vi "FRCts20_WebMethods_Convert_Teams.vi"(8 "error in (no error)":errorcluster, 11 "Team Out":T1) -> (0 "error out":errorcluster, 3 "Universe":T3)   [LabVIEW 2012, in "FRCts20_WebMethods.lvlib"]
uses:
  FRCts20_WebMethods.lvlib
  ESP Engine/source/VI Source/TypeDefs/FRCts20_EspEngine_Universe.ctl
  ESP Engine/source/VI Source/TypeDefs/FRCts20_EspEngine_Team.ctl
  Web Method Public Interface/FRCts20_WebMethods_ctl_singleTeam.ctl
  Web Method Public Interface/FRCts20_WebMethods_ctl_teamIdentifier.ctl
  Backend/source/VI Source/FRCts20_Backend_API/FRCts20_Backend_API_SW.ctl
  Web Method Public Interface/FRCts20_WebMethods_ctl_request.ctl
  Backend/source/VI Source/FRCts20_Backend_API/FRCts20_Backend_API_Status.ctl
  ESP Engine/source/VI Source/TypeDefs/FRCts20_EspEngine_Event.ctl
  Web Method Public Interface/FRCts20_WebMethods_ctl_singleEvent.ctl
  Backend/source/VI Source/FRCts20_Backend_API/FRCts20_Backend_API_TeamRoot.ctl
  Backend/source/VI Source/FRCts20_Backend_API/FRCts20_Backend_API.lvlib
  ESP Engine/source/VI Source/FRCts20_EspEngine.lvlib
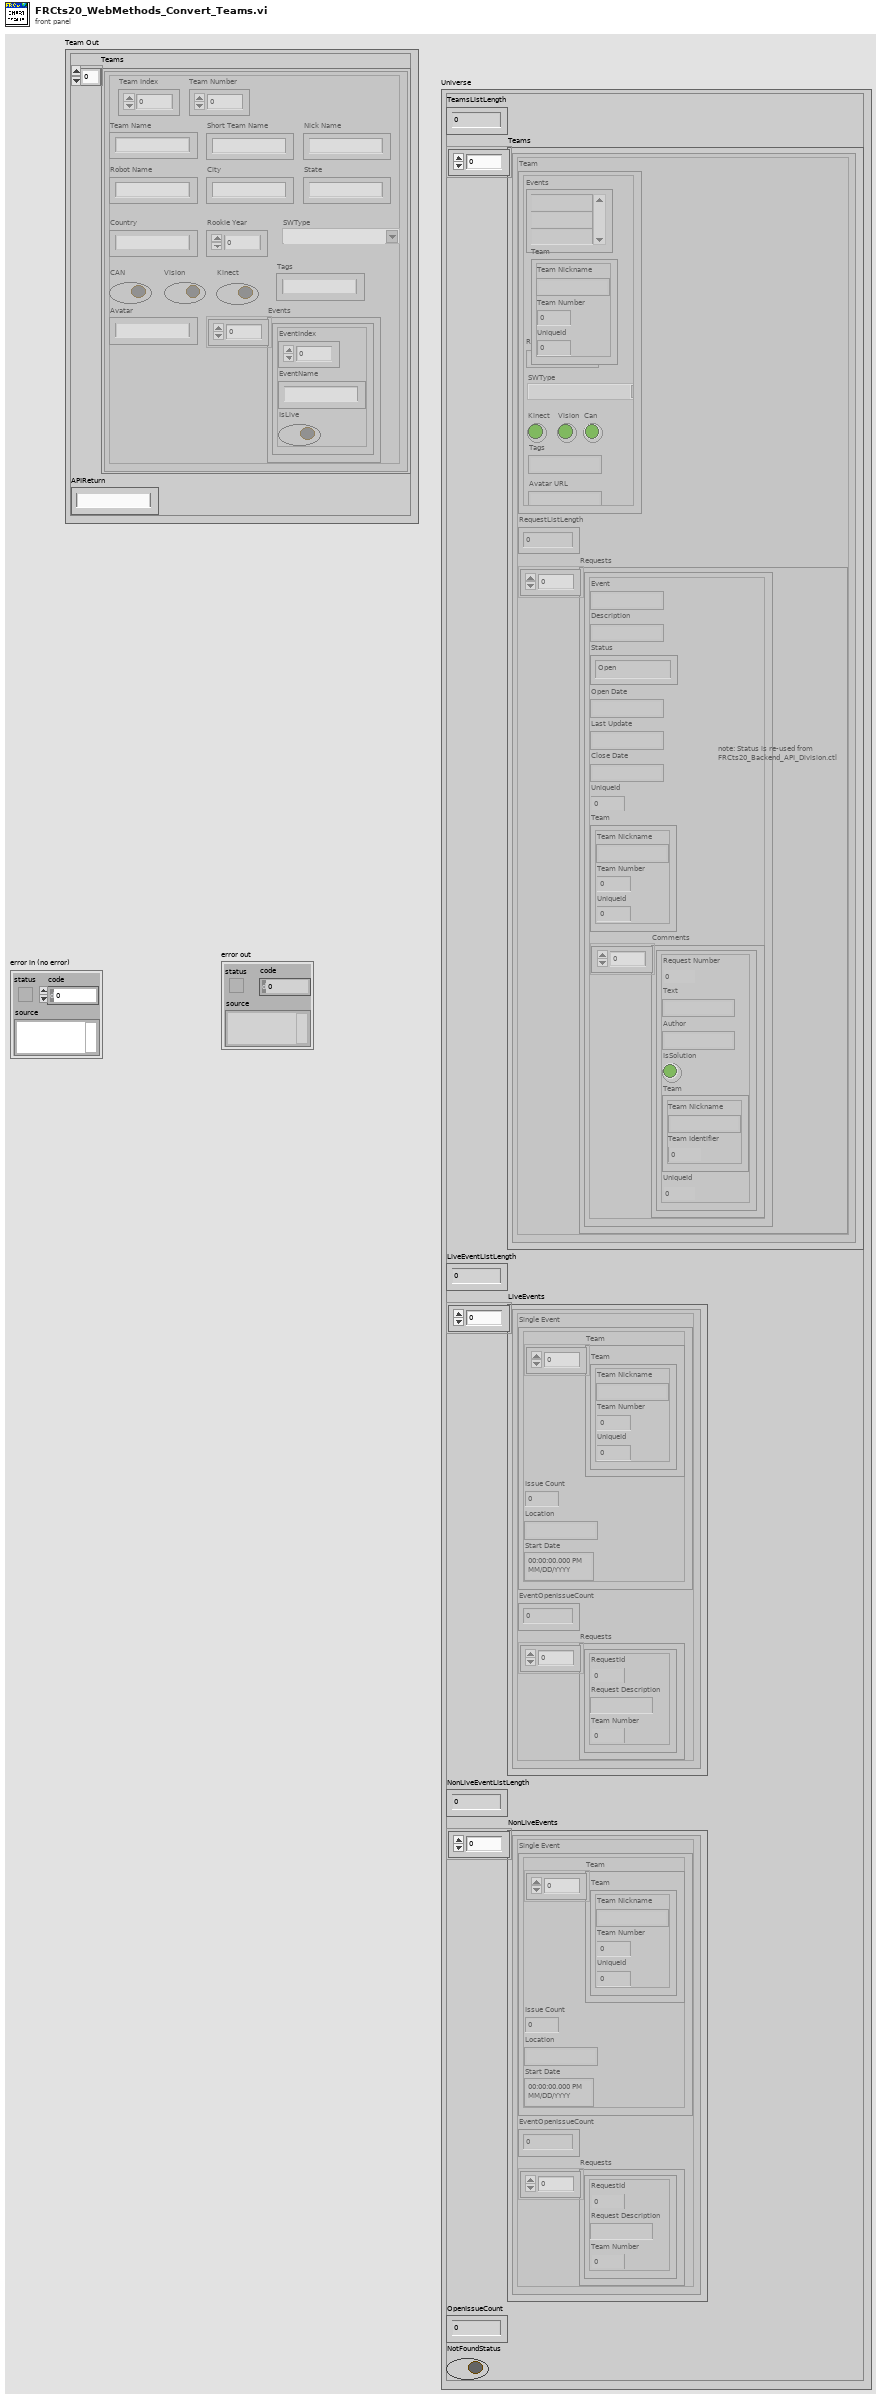
[diagram p1: front panel]
types:
  T1 = typedef "FRCts20_Backend_API.lvlib/FRCts20_Backend_API_TeamRoot.ctl" = cluster{"Teams":cluster{"Team Index":u32, "Team Number":u32, "Team Name":string, "Short Team Name":string, "Nick Name":string, "Robot Name":string, "City":string, "State":string, "Country":string, "Rookie Year":u32, "SWType":T2, "CAN":bool, "Vision":bool, "Kinect":bool, "Tags":string, "Avatar":string, "Events":cluster{"EventIndex":u32, "EventName":string, "IsLive":bool}[]}[], "APIReturn":string}
  T2 = typedef "FRCts20_Backend_API.lvlib/FRCts20_Backend_API_SW.ctl" = string
  T3 = typedef "FRCts20_EspEngine.lvlib/FRCts20_EspEngine_Universe.ctl" = cluster{"TeamsListLength":i16, "Teams":T4[], "LiveEventListLength":i16, "LiveEvents":T9[], "NonLiveEventListLength":i16, "NonLiveEvents":T9[], "OpenIssueCount":i16, "NotFoundStatus":bool}
  T4 = typedef "FRCts20_EspEngine.lvlib/FRCts20_EspEngine_Team.ctl" = cluster{"Team":T5, "RequestListLength":i16, "Requests":T7[]}
  T5 = typedef "FRCts20_WebMethods.lvlib/FRCts20_WebMethods_ctl_singleTeam.ctl" = cluster{"Events":string[], "Robot Name":string, "Kinect":bool, "Vision":bool, "Can":bool, "Tags":string, "Avatar URL":string, "Team":T6, "SWType":T2}
  T6 = typedef "FRCts20_WebMethods.lvlib/FRCts20_WebMethods_ctl_teamIdentifier.ctl" = cluster{"Team Nickname":string, "Team Number ":u32, "UniqueId":u32}
  T7 = typedef "FRCts20_WebMethods.lvlib/FRCts20_WebMethods_ctl_request.ctl" = cluster{"Event":string, "Description":string, "Status":T8, "Open Date":string, "Last Update":string, "Close Date":string, "UniqueId":i32, "Team":cluster{"Team Nickname":string, "Team Number ":i32, "UniqueId":i32}, "Comments":cluster{"Request Number":dbl, "Text":string, "Author":string, "IsSolution":bool, "Team":cluster{"Team Nickname":string, "Team Identifier ":dbl}, "UniqueId":i32}[]}
  T8 = typedef "FRCts20_Backend_API.lvlib/FRCts20_Backend_API_Status.ctl" = enum16{"Open", "In Work", "Closed"}
  T9 = typedef "FRCts20_EspEngine.lvlib/FRCts20_EspEngine_Event.ctl" = cluster{"Single Event":T10, "EventOpenIssueCount":i16, "Requests":cluster{"RequestId":i32, "Request Description":string, "Team Number":i32}[]}
  T10 = typedef "FRCts20_WebMethods.lvlib/FRCts20_WebMethods_ctl_singleEvent.ctl" = cluster{"Team":T6[], "Issue Count":i32, "Location":string, "Start Date ":timestamp}
  T11 = cluster{"Team Index":u32, "Team Number":u32, "Team Name":string, "Short Team Name":string, "Nick Name":string, "Robot Name":string, "City":string, "State":string, "Country":string, "Rookie Year":u32, "SWType":T2, "CAN":bool, "Vision":bool, "Kinect":bool, "Tags":string, "Avatar":string, "Events":cluster{"EventIndex":u32, "EventName":string, "IsLive":bool}[]}[]
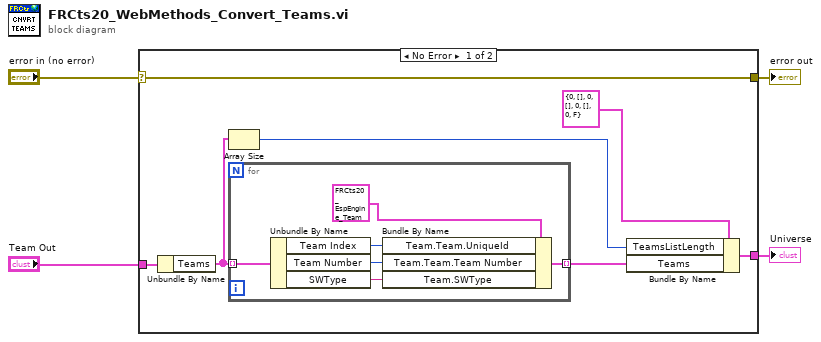
[diagram p0: block diagram]
diagram:
  n1 = case shown="No Error" "error in (no error)" {
    selector: "error in (no error)" -> [w5 w18]
    tunnel: [w5 w18] -> w4
    tunnel: "Team Out" -> [w7 _]
    tunnel: [w6 _] -> w1
    frame No Error {
      n2 = Unbundle By Name(w7) -> ("Teams"=w10:T11)
      n3 = Array Size(array=w10) -> (size(s)=w9:i32)
      n4 = for {
        tunnel: w10 -> [w16] mode=indexing
        tunnel: [w12] -> w8 mode=indexing
        n5 = Unbundle By Name(w16) -> ("Team Index"=w13:u32, "Team Number"=w14:u32, "SWType"=w15:T2)
        n6 = Bundle By Name(cluster=T4 {"Team"={"Events"=[], "Robot Name"="", "Kinect"=FALSE, "Vision"=FALSE, "Can"=FALSE, "Tags"="", "Avatar URL"="", "Team"={"Team Nickname"="", "Team Number "=0, "UniqueId"=0}, "SWType"=""}, "RequestListLength"=0, "Requests"=[]} ("Team"), "Team.Team.UniqueId"=w13, "Team.Team.Team Number"=w14, "Team.SWType"=w15) -> (w12:T4)
      }
      n7 = Bundle By Name(cluster=T3 {"TeamsListLength"=0, "Teams"=[], "LiveEventListLength"=0, "LiveEvents"=[], "NonLiveEventListLength"=0, "NonLiveEvents"=[], "OpenIssueCount"=0, "NotFoundStatus"=FALSE} ("Universe"), "TeamsListLength"=w9, "Teams"=w8) -> (w6:T3)
    }
    frame Error {
    }
  }
  "Universe" <- w1
  "error out" <- w4
